vi "old_HWGlobalsToObject.vi"(7 "Select Layout":refnum<vi>, 8 "error in (no error)":errorcluster, 10 "DDS Device":T1, 11 "DDS in":refnum<class "DDS.lvclass">) -> (0 "error out":errorcluster, 3 "DDS out":refnum<class "DDS.lvclass">)   [LabVIEW 2013, in "DDS.lvclass"]
uses:
  DDS.lvclass
  DDS.lvclass/DDS.ctl
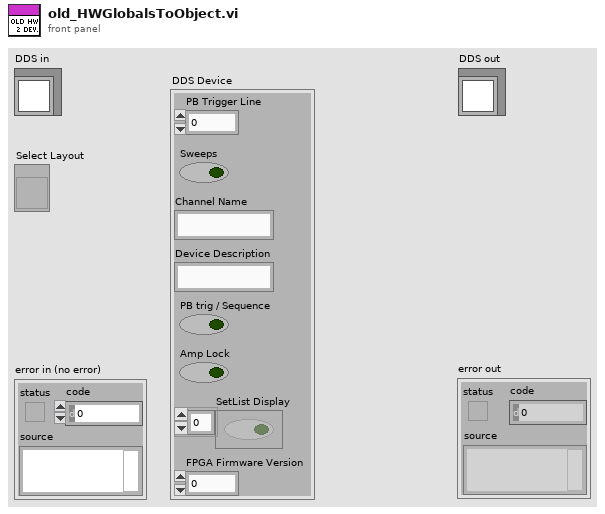
[diagram p1: front panel]
types:
  T1 = cluster{"PB Trigger Line":u16, "Sweeps":bool, "Channel Name":string, "Device Description":string, "PB trig / Sequence":bool, "Amp Lock":bool, "SetList Display":bool[], "FPGA Firmware Version":dbl}
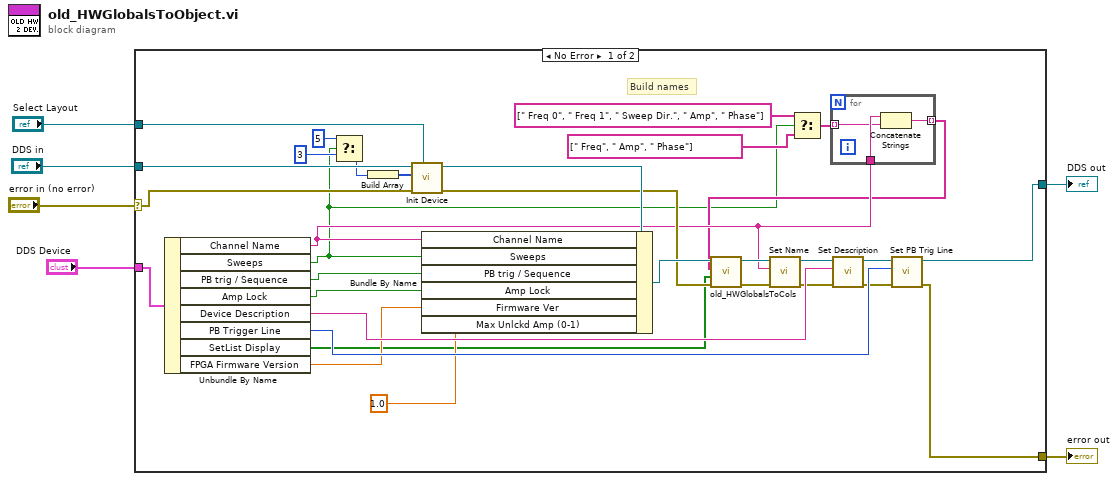
[diagram p0: block diagram]
diagram:
  n1 = case shown="No Error" "error in (no error)" {
    selector: "error in (no error)" -> [w24 w43]
    tunnel: [w31 w43] -> w5
    tunnel: [w30 w42] -> w3
    tunnel: "DDS in" -> [w25 w42]
    tunnel: "DDS Device" -> [w38 _]
    tunnel: "Select Layout" -> [w23 _]
    frame No Error {
      # "Build names"
      n2 = Unbundle By Name(w38) -> ("Channel Name"=w11:string, "Sweeps"=w7:bool, "PB trig / Sequence"=w37:bool, "Amp Lock"=w36:bool, "Device Description"=w35:string, "PB Trigger Line"=w33:u16, "SetList Display"=w14:bool[], "FPGA Firmware Version"=w27:dbl)
      n3 = Select(t=5 ("size(s)"), s=w7, f=3) -> (s? t:f=w22:i32)
      n4 = Build Array(w22) -> (w20:i32[])
      n5 = call-dynamic "Init Device.vi"("Layout Ref"=w23, "error in (no error)"=w24, "Chan# Array"=w20, "DDS in"=w25) -> ("error out"=w15:errorcluster, "DDS out"=w17:refnum<class "DDS.lvclass">)  [unwired: 6 in]
      n6 = Bundle By Name(cluster=w17, "Channel Name"=w11, "Sweeps"=w7, "PB trig / Sequence"=w37, "Amp Lock"=w36, "Firmware Ver"=w27, "Max Unlckd Amp (0-1)"=1.0 ("Hardware Limits.Max Unlckd Amp (0-1)")) -> (w16:refnum<class "DDS.lvclass">)
      n7 = Select(t=string[] [" Freq 0", " Freq 1", " Sweep Dir.", " Amp", " Phase"], s=w7, f=string[] [" Freq", " Amp", " Phase"]) -> (s? t:f=w12:string[])
      n8 = for {
        tunnel: w12 -> [w40] mode=indexing
        tunnel: w11 -> [w41]
        tunnel: [w39] -> w10 mode=indexing
        n9 = Concatenate Strings(w41, w40) -> (w39:string)
      }
      n10 = call-dynamic "old_HWGlobalsToCols.vi"("error in (no error)"=w15, "SetList Display"=w14, "Column Names"=w10, "Device in"=w16) -> ("error out"=w18:errorcluster, "Device out"=w13:refnum<class "DDS.lvclass">)  [unwired: 6 in]
      n11 = call-dynamic "Set Name.vi"("error in (no error)"=w18, "Name"=w11, "Device in"=w13) -> ("error out"=w28:errorcluster, "Device out"=w29:refnum<class "DDS.lvclass">)  [unwired: 7 in]
      n12 = call-dynamic "Set Description.vi"("error in (no error)"=w28, "Device Description"=w35, "Device in"=w29) -> ("error out"=w32:errorcluster, "Device out"=w34:refnum<class "DDS.lvclass">)  [unwired: 7 in]
      n13 = call-dynamic "Set PB Trig Line.vi"("error in (no error)"=w32, "PB Trigger Line"=w33, "Device in"=w34) -> ("error out"=w31:errorcluster, "Device out"=w30:refnum<class "DDS.lvclass">)  [unwired: 7 in]
    }
    frame Error {
    }
  }
  "error out" <- w5
  "DDS out" <- w3
